vi "conversionsGraph.vi"(7 "Array in":T2(array[cluster]), 8 "Numeric":dbl, 9 "T  (ºC)":dbl format="%.2g", 10 "RH  (%)":dbl format="%.2g", 11 "Ethanol (%)":dbl format="%.3g") -> (3 "Cluster":T1)   [LabVIEW 2019, in "DAQ.lvclass"]
uses:
  DAQ.lvclass
panel:
  out "error out":errorcluster
  in  "error in (no error)":errorcluster
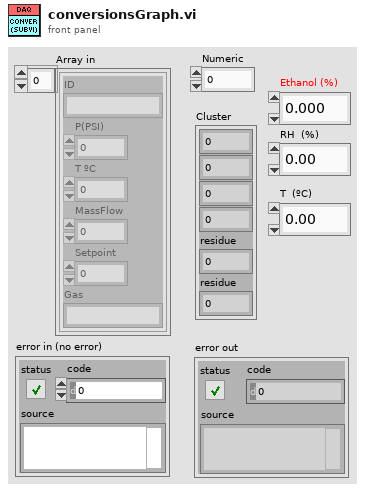
[diagram p1: front panel]
types:
  T1 = cluster{dbl, dbl, dbl, dbl, "residue":dbl, "residue":dbl}
  T2 = cluster{"ID":string, "P(PSI)":dbl, "T ºC":dbl, "MassFlow":dbl, "Setpoint":dbl, "Gas":string}[]
  T3 = cluster{"Numeric":dbl, "Ethanol (%)":dbl, "RH  (%) ":dbl, "T  (ºC) ":dbl, "residue":dbl, "residue":dbl}
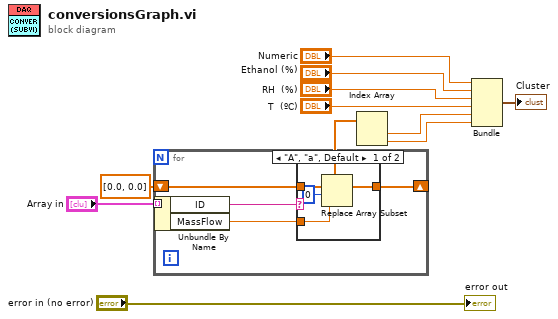
[diagram p0: block diagram]
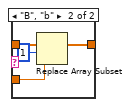
[diagram p2: hidden frame]
diagram:
  n1 = for {
    tunnel: "Array in" -> [w16] mode=indexing
    shift-right: [w13] -> w9
    shift-left: dbl[] [0.0, 0.0] -> [w14]
    n2 = Unbundle By Name(w16) -> ("ID"=w15:string, "MassFlow"=w12:dbl)
    n3 = case shown="\"A\", \"a\", Default" w15 {
      tunnel: [w20 w24] -> w13
      tunnel: w14 -> [w19 w23]
      tunnel: w12 -> [w18 w22]
      frame "A", "a", Default {
        n4 = Replace Array Subset(array=w19, new element=w18, index=0) -> (w20:dbl[])
      }
      frame "B", "b" {
        n5 = Replace Array Subset(array=w23, new element=w22, index=1) -> (w24:dbl[])
      }
    }
  }
  n6 = Index Array(array=w9) -> (element #1=w10:dbl, element #2=w11:dbl)  [unwired: 2 in]
  n7 = Bundle("Numeric"="Numeric", "Ethanol (%)"="Ethanol (%)", "RH  (%)"="RH  (%)", "T  (ºC)"="T  (ºC)", "residue"=w10, "residue"=w11) -> (→"Cluster":T3)  [unwired: 1 in]
  "error out" <- "error in (no error)"
